vi "writeCRC.vi"(8 "error in (no error)":errorcluster, 10 "Length":i32, 11 "ModbusBuffer in":refnum<class "ModbusBuffer.lvclass">) -> (0 "error out":errorcluster, 3 "ModbusBuffer out":refnum<class "ModbusBuffer.lvclass">)   [LabVIEW 2016, in "RTModbus.lvlib" / "ModbusBuffer.lvclass"]
uses:
  ModbusBuffer.lvclass
  ModbusBuffer.lvclass/ModbusBuffer.ctl
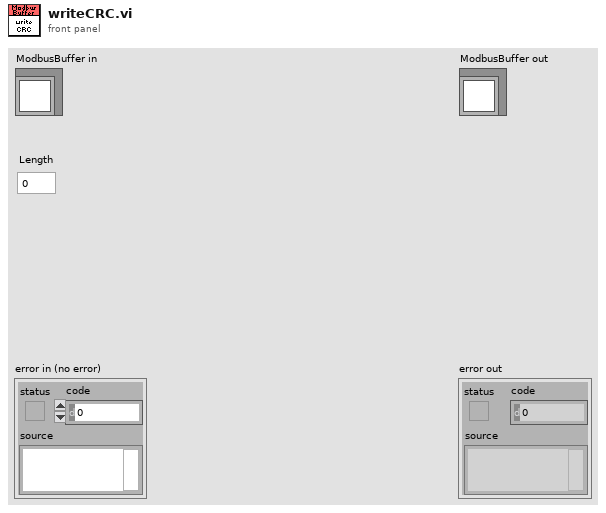
[diagram p1: front panel]
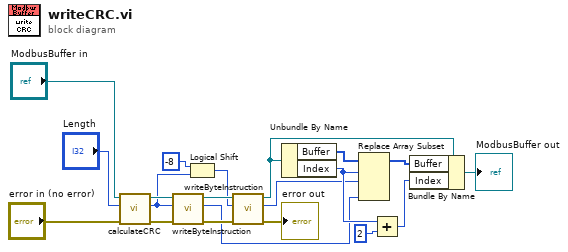
[diagram p0: block diagram]
diagram:
  n1 = call "calculateCRC.vi"("error in (no error)"="error in (no error)", "Length"="Length", "ModbusBuffer in"="ModbusBuffer in") -> ("error out"=w5:errorcluster, "CRC"=w3:u16, "ModbusBuffer out"=w7:refnum<class "ModbusBuffer.lvclass">)  [unwired: 6 in]
  n2 = call "writeByteInstruction.vi"("error in (no error)"=w5, "Input"=w3, "ModbusBuffer in"=w7) -> ("error out"=w14:errorcluster, "Output"=w2:u16, "ModbusBuffer out"=w16:refnum<class "ModbusBuffer.lvclass">)  [unwired: 6 in]
  n3 = Logical Shift(y=i16 -8, x=w3) -> (x << y=w15:u16)
  n4 = call "writeByteInstruction.vi"("error in (no error)"=w14, "Input"=w15, "ModbusBuffer in"=w16) -> ("error out"=→"error out":errorcluster, "Output"=w1:u16, "ModbusBuffer out"=w13:refnum<class "ModbusBuffer.lvclass">)  [unwired: 6 in]
  n5 = Unbundle By Name(w13) -> ("Buffer"=w11:u16[], "Index"=w10:i32)
  n6 = Replace Array Subset(array=w11, new element #1=w1, index #1=w10, new element #2=w2) -> (w17:u16[])  [unwired: 1 in]
  n7 = Add(x=w10, y=2) -> (x+y=w19:i32)
  n8 = Bundle By Name(cluster=w13, "Buffer"=w17, "Index"=w19) -> (→"ModbusBuffer out":refnum<class "ModbusBuffer.lvclass">)
